vi "Pockels Cal-Wizard window cleanup.vi"(8 "error in (no error)":errorcluster) -> ()   [LabVIEW 2020]
uses:
  Globals/gl_Calibration globals.vi
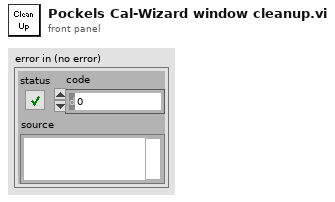
[diagram p1: front panel]
types:
  T1 = typedef "Pre-AOL Z wizard refs.ctl" = cluster{"VI's reference":refnum<vi>, "Calibration Mode":refnum<vi>, "Cal points":refnum<vi>, "Channel Selector":refnum<vi>, "Message":refnum<vi>, "Back":refnum<vi>, "Next":refnum<vi>, "Power meter AI":refnum<vi>, "2D Picture":refnum<vi>, "Note":refnum<vi>}
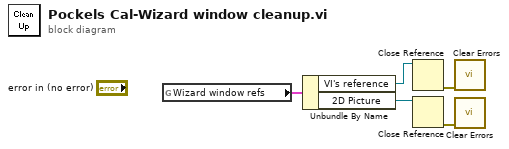
[diagram p0: block diagram]
diagram:
  n1 = global read "gl_Calibration globals.vi" "Wizard window refs"() -> (w5:T1)
  n2 = Unbundle By Name(w5) -> ("VI's reference"=w3:refnum<vi>, "2D Picture"=w4:refnum<vi>)
  n3 = Close Reference(reference=w3) -> (error out=w1:errorcluster)  [unwired: 1 in]
  n4 = Close Reference(reference=w4) -> (error out=w2:errorcluster)  [unwired: 1 in]
  n5 = call <vilib>:"Clear Errors.vi"("error in (no error)"=w1) -> ()  [unwired: 5 in, 2 out]
  n6 = call <vilib>:"Clear Errors.vi"("error in (no error)"=w2) -> ()  [unwired: 5 in, 2 out]
